vi "Sawtooth generation with curved edges.vi"() -> ()   [LabVIEW 2020]
uses:
  <vilib>/Analysis/1siggen.llb/Ramp Pattern by Samples.vi
  <vilib>/DAQmx/write.llb/DAQmx Write (Analog 1D Wfm NChan NSamp).vi
  <vilib>/DAQmx/create/channels.llb/DAQmx Create Channel (AO-Voltage-Basic).vi
  <vilib>/DAQmx/configure/timing.llb/DAQmx Timing (Use Waveform).vi
  <vilib>/DAQmx/miscellaneous.llb/DAQmx Fill In Error Info.vi
  <vilib>/Analysis/NI_AALBase.lvlib
  <vilib>/measure/NI_MABase.lvlib
panel:
  out "output waveform":waveform(dbl)={"t0"=timestamp(0 s since 1904-01-01), "dt"=0.001, "Y"=array[1000 elements]}
  out "Waveform Graph 4":waveform(dbl)[](graph)=[{"t0"=timestamp(0 s since 1904-01-01), "dt"=0.001, "Y"=array[1000 elements]}, {"t0"=timestamp(0 s since 1904-01-01), "dt"=0.001, "Y"=array[1000 elements]}]
  out "# Samples written per channel 2":u32=1000
  in  "Stop 2":bool
  out "Waveform Graph 3":waveform(dbl)[](graph)=[{"t0"=timestamp(0 s since 1904-01-01), "dt"=0.001, "Y"=array[1000 elements]}, {"t0"=timestamp(0 s since 1904-01-01), "dt"=0.001, "Y"=array[1000 elements]}]
  in  "Sawtooth Offset":dbl=0.03 format="%.2p"
  in  "Camera trigger delay (degrees)":dbl=-175.0 format="%.2p"
  in  "Exposure time (ms)":dbl=1000.0
  out "# Samples written per channel":u32=1000
  in  "Stop":bool
  in  "1 fps?":bool=TRUE
  in  "10 fps?":bool
  in  "Sawtooth Amplitude":dbl=0.455
  # "1. Turn on desired frame rate\n2. Run VI"
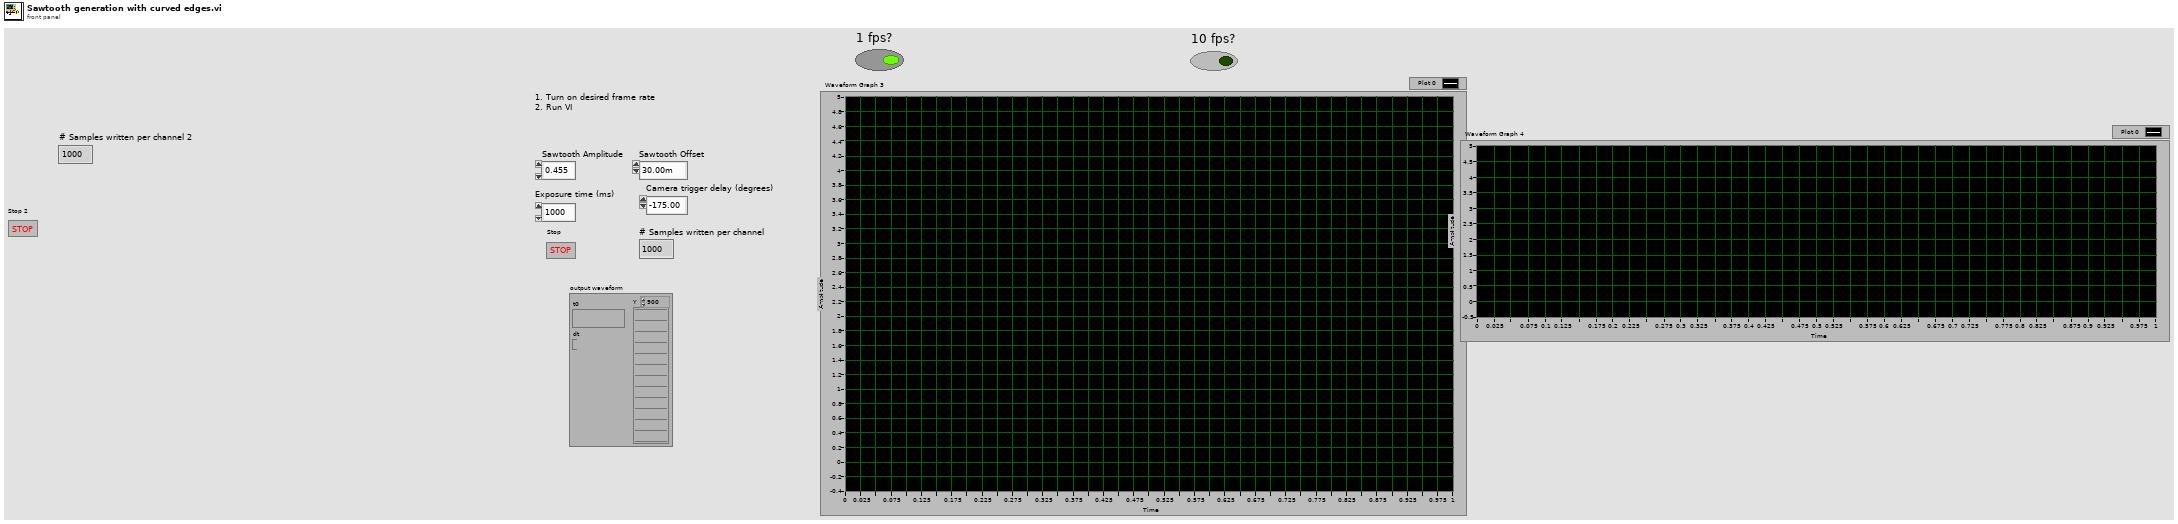
[diagram p1: front panel]
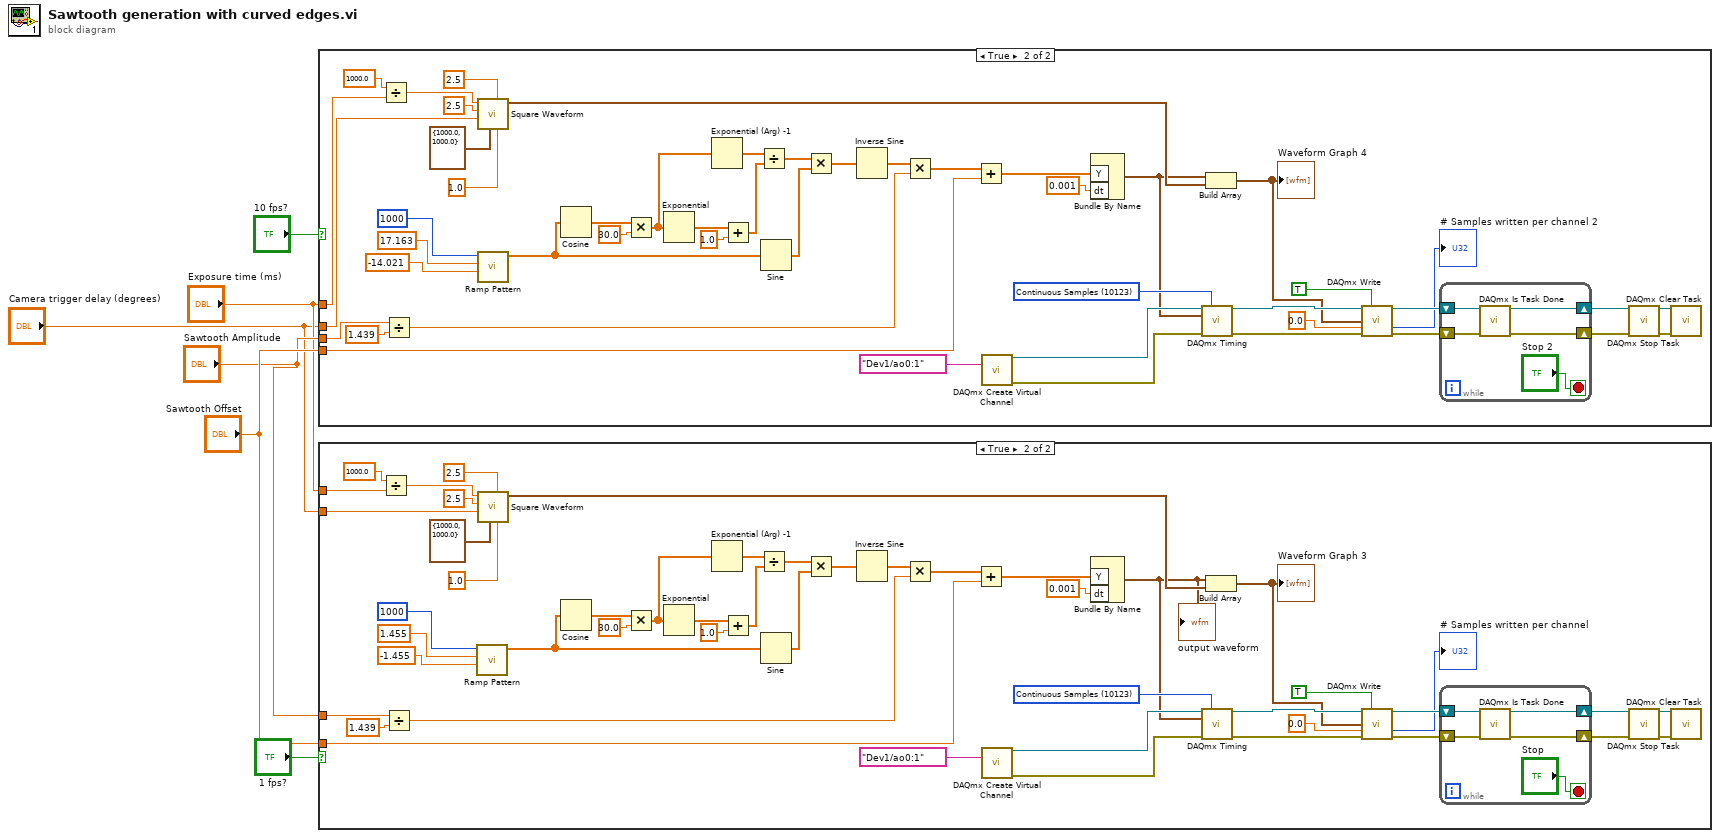
[diagram p0: block diagram]
diagram:
  n1 = case shown="True" "10 fps?" {
    tunnel: "Sawtooth Offset" -> [_ w9]
    tunnel: "Sawtooth Amplitude" -> [_ w50]
    tunnel: "Exposure time (ms)" -> [_ w8]
    tunnel: "Camera trigger delay (degrees)" -> [_ w7]
    frame False {
    }
    frame True {
      w44 = 10123 items=["Finite Samples"=10178, "Continuous Samples"=10123, "Hardware Timed Single Point"=12522] ("sample mode")
      n2 = Divide(x=1000.0, y=w8) -> (x/y=w27:dbl)
      n3 = Divide(x=w50, y=1.439) -> (x/y=w10:dbl)
      n4 = call <vilib>:"Square Waveform.vi"("duty cycle (%)"=1.0, "offset"=2.5, "sampling info"=cluster{"Fs":dbl, "#s":dbl} {"Fs"=1000.0, "#s"=1000.0}, "phase"=w7, "amplitude"=2.5, "frequency"=w27) -> ("signal out"=w30:waveform(dbl))  [unwired: 4 in, 1 out]
      n5 = call-poly <vilib>:"Ramp Pattern.vi"("start"=-14.021, "end"=17.163, "samples"=1000) -> ("Ramp Pattern"=w11:dbl[])  [unwired: 7 in, 1 out]
      n6 = Cosine(x=w11) -> (cos(x)=w25:dbl[])
      n7 = Multiply(x=w25, y=30.0) -> (x*y=w17:dbl[])
      n8 = Exponential(1:w17) -> (0:w20:dbl[])
      n9 = Exponential (Arg) -1(1:w17) -> (0:w24:dbl[])
      n10 = Add(x=w20, y=1.0) -> (x+y=w18:dbl[])
      n11 = Divide(x=w24, y=w18) -> (x/y=w23:dbl[])
      n12 = Sine(x=w11) -> (sin(x)=w22:dbl[])
      n13 = Multiply(x=w23, y=w22) -> (x*y=w21:dbl[])
      n14 = Inverse Sine(1:w21) -> (0:w15:dbl[])
      n15 = Multiply(x=w15, y=w10) -> (x*y=w14:dbl[])
      n16 = Add(x=w14, y=w9) -> (x+y=w13:dbl[])
      n17 = call-poly <vilib>:"DAQmx Create Virtual Channel.vi"("physical channels"=tag "Dev1/ao0:1") -> ("task out"=w46:refnum<k21>, "error out"=w45:errorcluster)  [unwired: 13 in]
      n18 = Bundle By Name("Y"=w13, "dt"=0.001) -> (w12:waveform(dbl))  [unwired: 1 in]
      n19 = call-poly <vilib>:"DAQmx Timing.vi"("task/channels in"=w46, "sample mode"=w44, "waveform"=w12, "error in"=w45) -> ("task out"=w41:refnum<k21>, "error out"=w40:errorcluster)  [unwired: 10 in]
      n20 = Build Array(w12, w30) -> (w28:waveform(dbl)[])
      "Waveform Graph 4" <- w28
      n21 = call-poly <vilib>:"DAQmx Write.vi"("task/channels in"=w41, "auto start"=TRUE, "data"=w28, "timeout"=0.0, "error in"=w40) -> ("task out"=w42:refnum<k21>, "number of samples written per channel"=→"# Samples written per channel 2":u32, "error out"=w43:errorcluster)  [unwired: 8 in]
      n22 = while {
        shift-right: [w56] -> w38
        shift-left: w42 -> [w59]
        shift-right: [w57] -> w39
        shift-left: w43 -> [w58]
        stop <- "Stop 2" stop-if-true
        n23 = call <vilib>:"DAQmx Is Task Done.vi"("task/channels in"=w59, "error in"=w58) -> ("task out"=w56:refnum<k21>, "error out"=w57:errorcluster)  [unwired: 11 in, 1 out]
      }
      n24 = call <vilib>:"DAQmx Stop Task.vi"("task/channels in"=w38, "error in"=w39) -> ("task out"=w47:refnum<k21>, "error out"=w48:errorcluster)  [unwired: 12 in]
      n25 = call <vilib>:"DAQmx Clear Task.vi"("task in"=w47, "error in"=w48) -> ()  [unwired: 13 in, 1 out]
    }
  }
  n26 = case shown="True" "1 fps?" {
    tunnel: "Sawtooth Offset" -> [_ w84]
    tunnel: "Sawtooth Amplitude" -> [_ w83]
    tunnel: "Exposure time (ms)" -> [_ w61]
    tunnel: "Camera trigger delay (degrees)" -> [_ w60]
    frame False {
    }
    frame True {
      w102 = 10123 items=["Finite Samples"=10178, "Continuous Samples"=10123, "Hardware Timed Single Point"=12522] ("sample mode")
      n27 = Divide(x=1000.0, y=w61) -> (x/y=w85:dbl)
      n28 = Divide(x=w83, y=1.439) -> (x/y=w68:dbl)
      n29 = call-poly <vilib>:"Ramp Pattern.vi"("start"=-1.455, "end"=1.455, "samples"=1000) -> ("Ramp Pattern"=w65:dbl[])  [unwired: 7 in, 1 out]
      n30 = call <vilib>:"Square Waveform.vi"("duty cycle (%)"=1.0, "offset"=2.5, "sampling info"=cluster{"Fs":dbl, "#s":dbl} {"Fs"=1000.0, "#s"=1000.0}, "phase"=w60, "amplitude"=2.5, "frequency"=w85) -> ("signal out"=w88:waveform(dbl))  [unwired: 4 in, 1 out]
      n31 = Cosine(x=w65) -> (cos(x)=w78:dbl[])
      n32 = Multiply(x=w78, y=30.0) -> (x*y=w70:dbl[])
      n33 = Exponential(1:w70) -> (0:w73:dbl[])
      n34 = Exponential (Arg) -1(1:w70) -> (0:w77:dbl[])
      n35 = Add(x=w73, y=1.0) -> (x+y=w71:dbl[])
      n36 = Divide(x=w77, y=w71) -> (x/y=w76:dbl[])
      n37 = Sine(x=w65) -> (sin(x)=w75:dbl[])
      n38 = Multiply(x=w76, y=w75) -> (x*y=w74:dbl[])
      n39 = Inverse Sine(1:w74) -> (0:w67:dbl[])
      n40 = Multiply(x=w67, y=w68) -> (x*y=w64:dbl[])
      n41 = Add(x=w64, y=w84) -> (x+y=w63:dbl[])
      n42 = call-poly <vilib>:"DAQmx Create Virtual Channel.vi"("physical channels"=tag "Dev1/ao0:1") -> ("task out"=w104:refnum<k21>, "error out"=w103:errorcluster)  [unwired: 13 in]
      n43 = Bundle By Name("Y"=w63, "dt"=0.001) -> (w62:waveform(dbl))  [unwired: 1 in]
      "output waveform" <- w62
      n44 = call-poly <vilib>:"DAQmx Timing.vi"("task/channels in"=w104, "sample mode"=w102, "waveform"=w62, "error in"=w103) -> ("task out"=w99:refnum<k21>, "error out"=w98:errorcluster)  [unwired: 10 in]
      n45 = Build Array(w62, w88) -> (w86:waveform(dbl)[])
      "Waveform Graph 3" <- w86
      n46 = call-poly <vilib>:"DAQmx Write.vi"("task/channels in"=w99, "auto start"=TRUE, "data"=w86, "timeout"=0.0, "error in"=w98) -> ("task out"=w100:refnum<k21>, "number of samples written per channel"=→"# Samples written per channel":u32, "error out"=w101:errorcluster)  [unwired: 8 in]
      n47 = while {
        shift-right: [w109] -> w96
        shift-left: w100 -> [w112]
        shift-right: [w110] -> w97
        shift-left: w101 -> [w111]
        stop <- "Stop" stop-if-true
        n48 = call <vilib>:"DAQmx Is Task Done.vi"("task/channels in"=w112, "error in"=w111) -> ("task out"=w109:refnum<k21>, "error out"=w110:errorcluster)  [unwired: 11 in, 1 out]
      }
      n49 = call <vilib>:"DAQmx Stop Task.vi"("task/channels in"=w96, "error in"=w97) -> ("task out"=w105:refnum<k21>, "error out"=w106:errorcluster)  [unwired: 12 in]
      n50 = call <vilib>:"DAQmx Clear Task.vi"("task in"=w105, "error in"=w106) -> ()  [unwired: 13 in, 1 out]
    }
  }
